vi "Error Type.vi"(5 "Error Type":T1(ring)) -> (2 "Log":string)   [LabVIEW 2014]
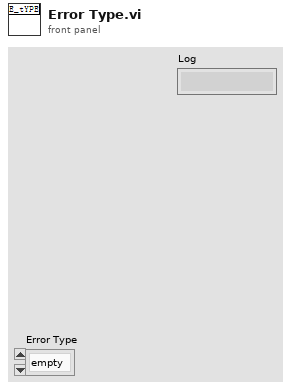
[diagram p1: front panel]
types:
  T1 = enum16{"empty", "Serial Error", "op Read", "IP TCP", "Other"}
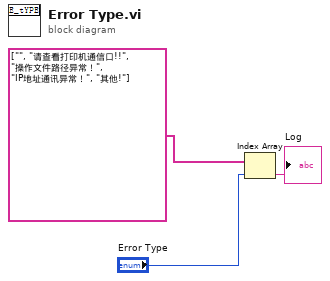
[diagram p0: block diagram]
diagram:
  n1 = Index Array(array=string[] ["", "请查看打印机通信口!!", "操作文件路径异常！", "IP地址通讯异常！", "其他!"], index="Error Type") -> (element=→"Log":string)
